vi "createInstance.vi"(8 "error in (no error)":errorcluster, 11 "IInstance in":refnum<class "IInstance.lvclass">) -> (0 "error out":errorcluster, 3 "IInstance out":refnum<class "IInstance.lvclass">)   [LabVIEW 2022 SP3, in "openDAQ.lvlib" / "daqUtils.lvlib"]
uses:
  daqUtils.lvlib
  IInstanceBuilder/IInstanceBuilder.lvclass
  IInstance/IInstance.lvclass
  openDAQ.lvlib
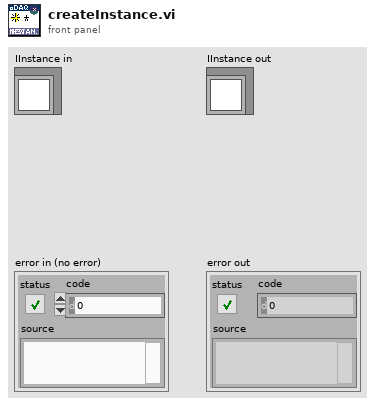
[diagram p1: front panel]
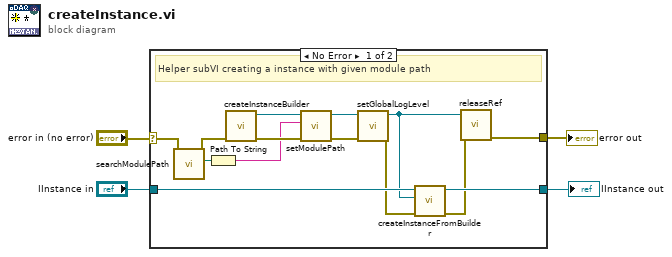
[diagram p0: block diagram]
diagram:
  n1 = case shown="No Error" "error in (no error)" {
    selector: "error in (no error)" -> [w6 w20]
    tunnel: "IInstance in" -> [w18 w19]
    tunnel: [w17 w19] -> w3
    tunnel: [w16 w20] -> w2
    frame No Error {
      # "Helper subVI creating a instance with given module path"
      n2 = call "searchModulePath.vi"("error in (no error)"=w6) -> ("error out"=w5:errorcluster, "module path out"=w8:path)  [unwired: 9 in]
      n3 = Path To String(path=w8) -> (string=w7:string)
      n4 = call "createInstanceBuilder.vi"("error in (no error)"=w5) -> ("error out"=w9:errorcluster, "IInstanceBuilder out"=w10:refnum<class "IInstanceBuilder.lvclass">)  [unwired: 9 in]
      n5 = call "setModulePath.vi"("error in (no error)"=w9, "modulePathStr"=w7, "IInstanceBuilder in"=w10) -> ("error out"=w11:errorcluster, "IInstanceBuilder out"=w12:refnum<class "IInstanceBuilder.lvclass">)  [unwired: 7 in]
      n6 = call "setGlobalLogLevel.vi"("error in (no error)"=w11, "IInstanceBuilder in"=w12) -> ("error out"=w13:errorcluster, "IInstanceBuilder out"=w15:refnum<class "IInstanceBuilder.lvclass">)  [unwired: 8 in]
      n7 = call "createInstanceFromBuilder.vi"("error in (no error)"=w13, "IInstanceBuilder in"=w15, "IInstance in"=w18) -> ("error out"=w14:errorcluster, "IInstance out"=w17:refnum<class "IInstance.lvclass">)  [unwired: 7 in]
      n8 = call-dynamic "releaseRef.vi"("error in (no error)"=w14, "IBaseObject in"=w15) -> ("error out"=w16:errorcluster)  [unwired: 9 in]
    }
    frame Error {
    }
  }
  "IInstance out" <- w3
  "error out" <- w2
